vi "Delete.vi"(5 "Delete all found":bool, 6 "$Path or Item Name":string, 7 "error in (no error)":errorcluster, 9 "Offset":i32, 10 "JSON":string="{}") -> (0 "error out":errorcluster, 1 "<JSON> First Deleted Item":string, 2 "Number Deleted":i32, 3 "<JSON>":string caption="<JSON>With Item Deleted")   [LabVIEW 2017, in "JSONtext.lvlib"]
doc: "Deletes JSON item at the JSON Path specified. If \"Delete all found\" is True, will delete all items matching the path. Else will just delete the first found."
uses:
  JSONtext.lvlib
  Parsing/Parsing State.ctl
  support/Quote and Escape JSON string.vi
  Parsing/Advance past whitespace.vi
  support/quote and escape json string 2.vi
  Parsing/Path Notation End Name.vi
  Parsing/Parse Full Path or Item Name.vi
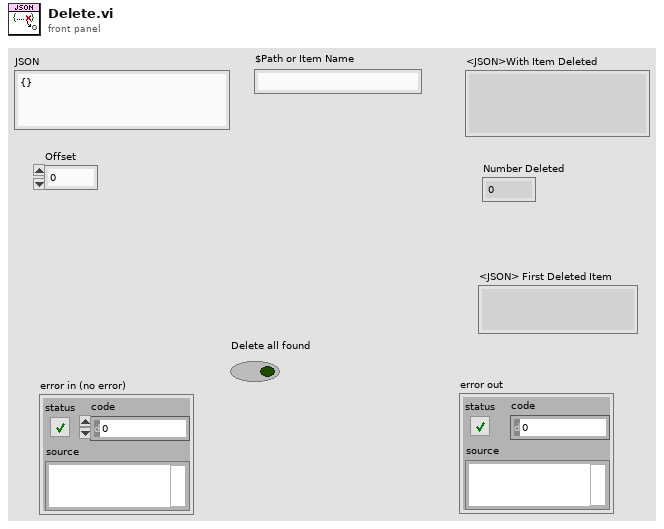
[diagram p1: front panel]
types:
  T1 = typedef "JSONtext.lvlib/Found Items.ctl" = cluster{"Item offset":i32, "Offset past Item":i32, "Name offset":i32, "Offset past Name":i32, "Found":bool, "Item Type":T2, "Item Index":i32}
  T2 = typedef "JSONtext.lvlib/Parsing State.ctl" = enum16{"Parser Error", "Object", "Array", "String", "Number/Other", "Leading Whitespace", "Object end", "Array end", "Value end"}
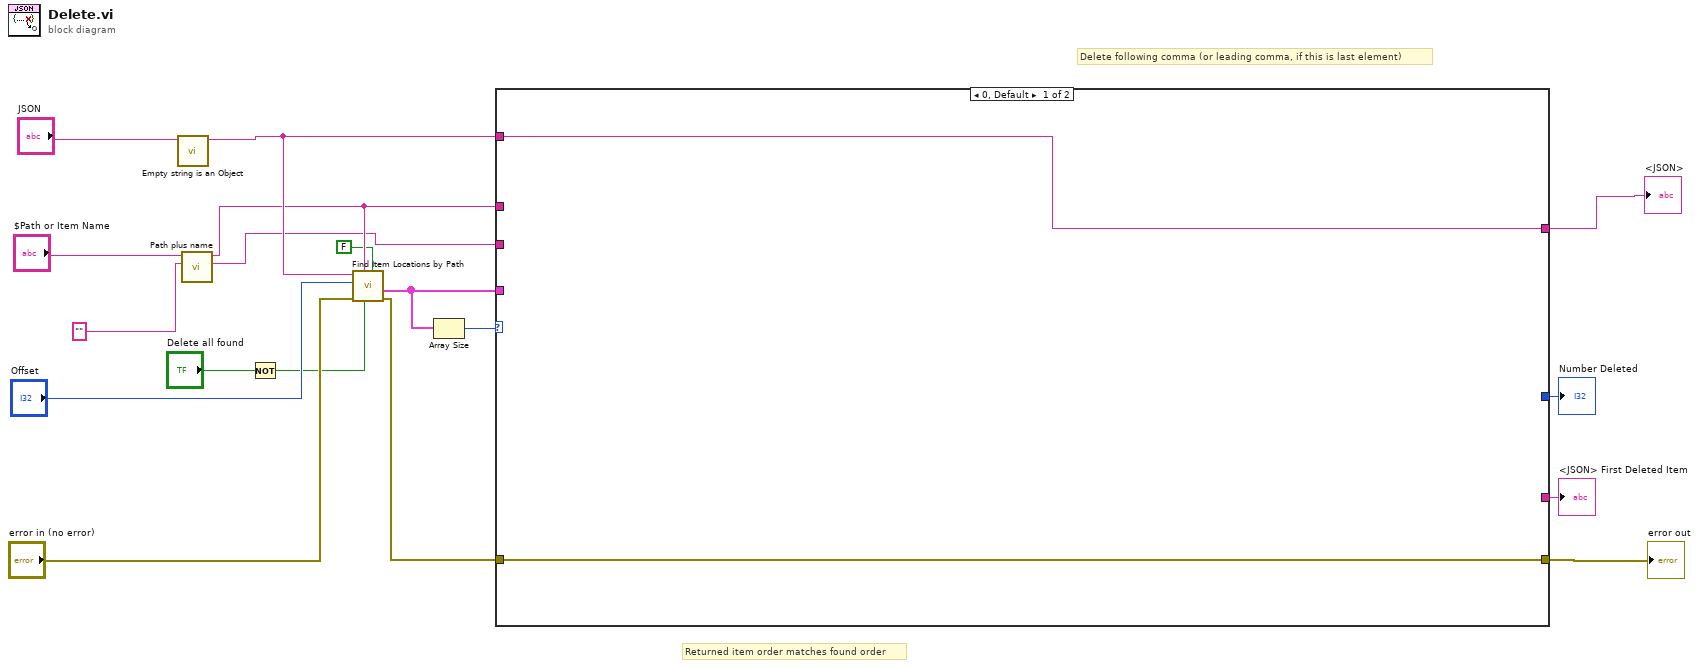
[diagram p0: block diagram]
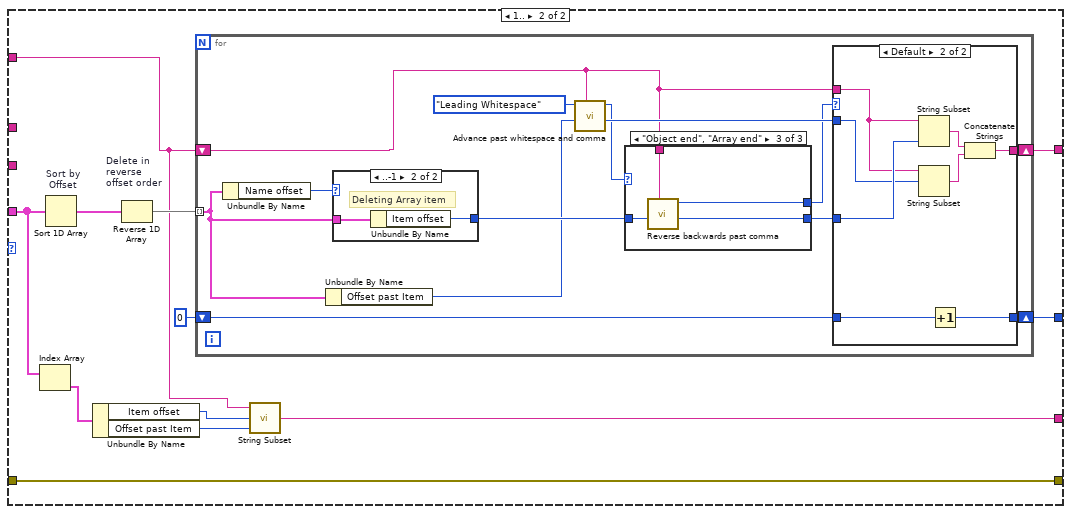
[diagram p2: hidden frame]
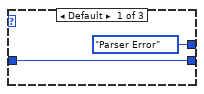
[diagram p4: hidden frame]
diagram:
  # "Returned item order matches found order"
  # "Delete following comma (or leading comma, if this is last element)"
  n1 = call "Empty string is an Object.vi"("JSON Input"="JSON") -> ("<JSON>Object"=w13:string)  [unwired: 10 in]
  n2 = call "Path plus name.vi"("Item Name"="", "Object (or Item) Path"="$Path or Item Name") -> ("<JSON>End Name"=w9:string, "Relative Path or JSON-format name"=w10:string)  [unwired: 7 in, 1 out]
  n3 = Not(x="Delete all found") -> (.not. x?=w2:bool)
  n4 = call "Find Item Locations by Path.vi"("Insertion point if not found"=FALSE, "Only return first found"=w2, "Path"=w10, "error in (no error)"="error in (no error)", "Offset"="Offset", "JSON"=w13) -> ("error out"=w5:errorcluster, "Items"=w7:T1[])  [unwired: 4 in]
  n5 = Array Size(array=w7) -> (size(s)=w6:i32)
  n6 = case shown="0, Default" w6 {
    tunnel: [w20 w31] -> w18
    tunnel: w13 -> [w20 w22]
    tunnel: w7 -> [_ w24]
    tunnel: w9 -> [_ _]
    tunnel: w5 -> [w19 w32]
    tunnel: w10 -> [_ _]
    tunnel: [w19 w32] -> w15
    tunnel: [_ w27] -> w3
    tunnel: [_ w21] -> w1
    frame 0, Default {
    }
    frame 1.. {
      n7 = Index Array(array=w24) -> (element=w23:T1)  [unwired: 1 in]
      n8 = Sort 1D Array "Sort by\n Offset"(array=w24) -> (sorted array=w29:T1[])
      n9 = Unbundle By Name(w23) -> ("Item offset"=w26:i32, "Offset past Item"=w25:i32)
      n10 = Reverse 1D Array "Delete in \nreverse\noffset order"(array=w29) -> (reversed array=w30:T1[])
      n11 = for {
        tunnel: w30 -> [w37] mode=indexing
        shift-right: [w44] -> w31
        shift-left: w22 -> [w35]
        shift-right: [w34] -> w27
        shift-left: 0 -> [w33]
        n12 = Unbundle By Name(w37) -> ("Name offset"=w39:i32)
        n13 = Unbundle By Name(w37) -> ("Offset past Item"=w36:i32)
        n14 = case shown="..-1" w39 {
          selector: w39 -> [w46 _]
          tunnel: [w46 w48] -> w38
          tunnel: w37 -> [_ w47]
          frame 0.. {
            # "Deleting Object item"
          }
          frame ..-1 {
            # "Deleting Array item"
            n15 = Unbundle By Name(w47) -> ("Item offset"=w48:i32)
          }
        }
        n16 = call "Advance past whitespace and comma.vi"("JSON"=w35, "Offset"=w36, "State in"=Parsing_State."Leading Whitespace") -> ("Offset past match"=w45:i32, "State"=w42:T2)  [unwired: 7 in]
        n17 = case shown="\"Object end\", \"Array end\"" w42 {
          selector: w42 -> [_ w51 _]
          tunnel: w38 -> [w50 w52 w56]
          tunnel: [w50 w52 w55] -> w43
          tunnel: w35 -> [_ _ w54]
          tunnel: [Parsing_State."Parser Error" ("Parser State") w51 w53] -> w41
          frame Default {
          }
          frame "Object".."Number/Other" {
          }
          frame "Object end", "Array end" {
            n18 = call "Reverse backwards past comma.vi"("JSON"=w54, "Offset"=w56) -> ("Offset of first non-whitespace"=w55:i32, "Parser State"=w53:T2)  [unwired: 8 in]
          }
        }
        n19 = case shown="Default" w41 {
          tunnel: w35 -> [w58 w61]
          tunnel: w43 -> [_ w66]
          tunnel: w45 -> [_ w65]
          tunnel: [w58 w62] -> w44
          tunnel: [w57 w60] -> w34
          tunnel: w33 -> [w57 w59]
          frame "Parser Error" {
          }
          frame Default {
            n20 = String Subset(string=w61, length (rest)=w66) -> (substring=w64:string)  [unwired: 1 in]
            n21 = String Subset(string=w61, offset (0)=w65) -> (substring=w63:string)  [unwired: 1 in]
            n22 = Increment(x=w59) -> (x+1=w60:i32)
            n23 = Concatenate Strings(w64, w63) -> (w62:string)
          }
        }
      }
      n24 = call "String Subset.vi"("Offset past End"=w25, "Start offset"=w26, "JSON"=w22) -> ("substring"=w21:string)  [unwired: 2 in]
    }
  }
  "<JSON>" <- w18
  "error out" <- w15
  "Number Deleted" <- w3
  "<JSON> First Deleted Item" <- w1
